vi "Do.vi"(8 "error in (no error)":errorcluster, 10 "Actor In":refnum<class "Actor.lvclass">, 11 "Data Count Msg in":refnum<class "Data Count Msg.lvclass">) -> (0 "error out":errorcluster, 1 "Stop Actor":bool, 2 "Actor Out":refnum<class "Actor.lvclass">)   [LabVIEW 2022 SP3, in "Scratchpad.lvlib" / "Test 1.lvlib" / "Data Count Msg.lvclass"]
uses:
  Data Count Msg.lvclass
  Artifex/Actor/Actor.lvclass
  Data Count Msg.lvclass/Data Count Msg.ctl
  a618fff3-136c-4cf6-a3b9-575232d98459.vi
  Data Count Handler/Data Count Handler.lvclass
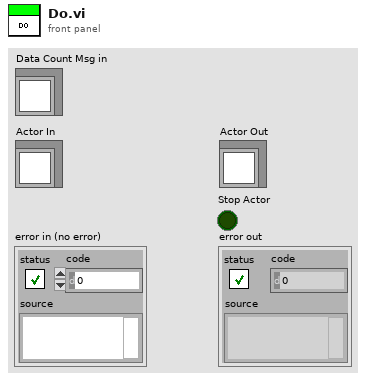
[diagram p1: front panel]
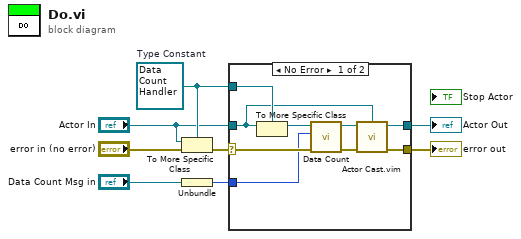
[diagram p0: block diagram]
diagram:
  w6 = refnum<class "Data Count Handler.lvclass"> refnum  # Type Constant
  n1 = To More Specific Class(target class=w6, reference="Actor In", error in="error in (no error)") -> (error out=w7:errorcluster)  [unwired: 1 out]
  n2 = Unbundle("Data Count Msg in") -> (w8:i32)
  n3 = case shown="No Error" w7 {
    selector: w7 -> [w17 w18]
    tunnel: [w13 w19] -> w2
    tunnel: [w10 w18] -> w1
    tunnel: w8 -> [w15 _]
    tunnel: w6 -> [w11 _]
    tunnel: "Actor In" -> [w9 w19]
    frame No Error {
      n4 = To More Specific Class(target class=w11, reference=w9) -> (specific class reference=w14:refnum<class "Data Count Handler.lvclass">)  [unwired: 1 in, 1 out]
      n5 = call "Data Count.vi"("error in (no error)"=w17, "Data Count"=w15, "Data Count Handler in"=w14) -> ("error out"=w12:errorcluster, "Data Count Handler out"=w16:refnum<class "Data Count Handler.lvclass">)  [unwired: 7 in]
      n6 = call "Actor Cast.vim"("Type"=w9, "Actor in"=w16, "error in (no error)"=w12) -> ("Actor out"=w13:refnum<class "Actor.lvclass">, "error out"=w10:errorcluster)  [unwired: 6 in]
    }
    frame Error {
    }
  }
  "error out" <- w1
  "Actor Out" <- w2
